vi "Configure Modules from Hardware.vi"() -> ()   [LabVIEW 2017, in "SLSC Switch Examples.lvlib"]
uses:
  SLSC Switch Examples.lvlib
  NationalInstruments.VeriStand.SystemDefinitionAPI
  SLSC Switch/Shared/Endpoint Configuration Cluster.ctl
  SLSC Switch/Shared/Endpoint Configuration Enum.ctl
  SLSC Switch/Scripting/SLSC Switch Scripting.lvlib
  SLSC Switch/Shared/SLSC Switch Shared.lvlib
panel:
  in  "SLSC Switch devices":refnum<k21>[](array[refnum])
  out "error out":errorcluster
  in  "error in (no error)":errorcluster
  in  "output system definition":path
  in  "input system definition":path
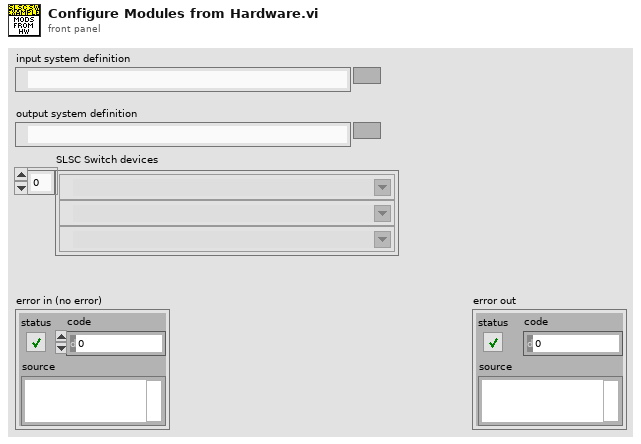
[diagram p1: front panel]
types:
  T1 = typedef "SLSC Switch Shared.lvlib/Endpoint Configuration Enum.ctl" = enum16{"Load", "Source", "Configuration"}
  T2 = typedef "SLSC Switch Shared.lvlib/Endpoint Configuration Cluster.ctl" = cluster{"Endpoint":string, "Configuration":T1}
  T3 = typedef "Custom Device API.lvlib/Custom Device Item Ref.ctl" = u64
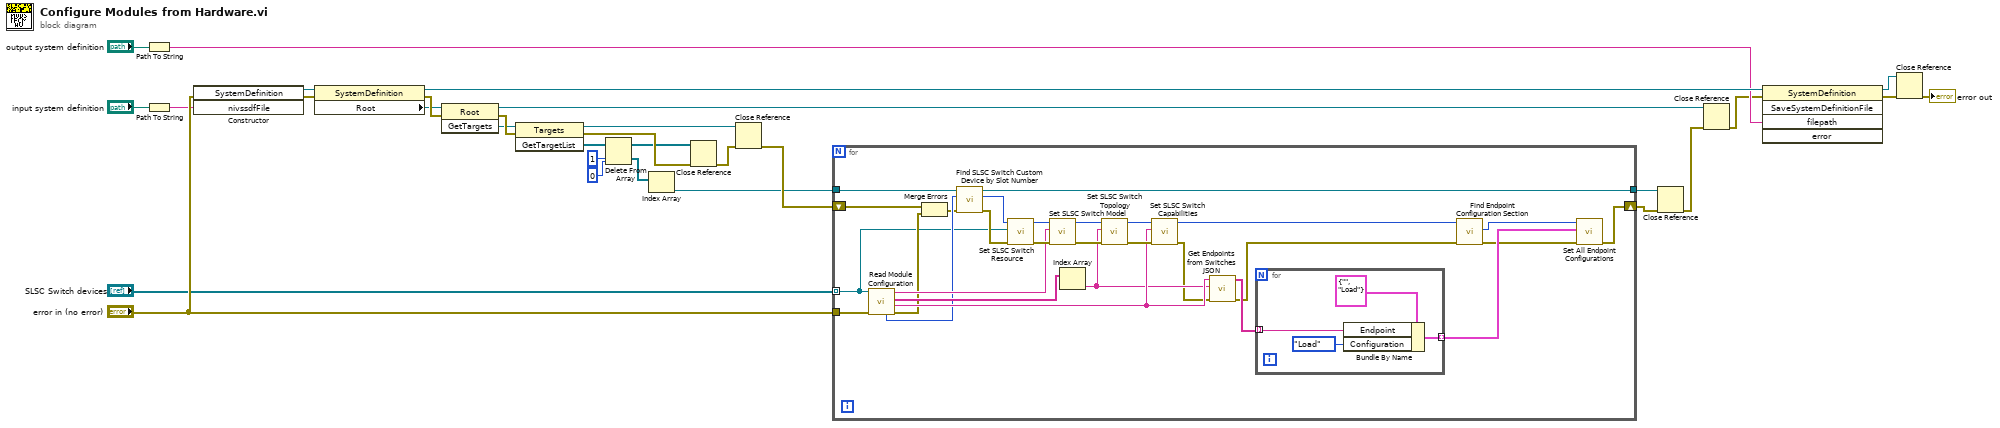
[diagram p0: block diagram]
diagram:
  n1 = Path To String(path="output system definition") -> (string=w16:string)
  n2 = Path To String(path="input system definition") -> (string=w8:string)
  n3 = constructor class="SystemDefinition"(error in="error in (no error)", "nivssdfFile"=w8) -> (reference out=w30:refnum<k24>, error out=w31:errorcluster)  [unwired: 2 in, 2 out]
  n4 = property class="SystemDefinition"(reference=w30, error in=w31) -> (reference out=w17:refnum<k24>, error out=w29:errorcluster, "Root"=w28:refnum<k24>)
  n5 = invoke class="Root" method="GetTargets"(reference=w28, error in=w29) -> (reference out=w13:refnum<k24>, error out=w27:errorcluster, "GetTargets"=w26:refnum<k24>)  [unwired: 1 in]
  n6 = invoke class="Targets" method="GetTargetList"(reference=w26, error in=w27) -> (reference out=w19:refnum<k24>, error out=w22:errorcluster, "GetTargetList"=w25:refnum<k24>[])  [unwired: 1 in]
  n7 = Delete From Array(array=w25, length=1, index=0) -> (deleted portion=w18:refnum<k24>[], array with subset deleted=w21:refnum<k24>[])
  n8 = Index Array(array=w18) -> (element=w5:refnum<k24>)  [unwired: 1 in]
  n9 = Close Reference(reference=w21, error in (no error)=w22) -> (error out=w20:errorcluster)
  n10 = Close Reference(reference=w19, error in (no error)=w20) -> (error out=w6:errorcluster)
  n11 = for {
    tunnel: "error in (no error)" -> [w46]
    tunnel: w5 -> [w44]
    tunnel: "SLSC Switch devices" -> [w34] mode=indexing
    shift-right: [w32] -> w1
    shift-left: w6 -> [w45]
    tunnel: [w33] -> w3
    n12 = call "Read Module Configuration.vi"("error in (no error)"=w46, "SLSC Device"=w34) -> ("error out"=w39:errorcluster, "switches json"=w51:string, "topologies"=w53:string[], "product name"=w57:string, "slot number"=w41:u32)  [unwired: 5 in]
    n13 = Merge Errors(w45, w39) -> (w40:errorcluster)
    n14 = call "Find SLSC Switch Custom Device by Slot Number.vi"("error in (no error)"=w40, "slot number"=w41, "Target in"=w44) -> ("error out"=w42:errorcluster, "SLSC Switch Custom Device Ref"=w43:T3, "Target out"=w33:refnum<k24>)  [unwired: 6 in]
    n15 = call "Set SLSC Switch Resource.vi"("error in (no error)"=w42, "Resource"=w34, "SLSC Switch Custom Device Ref in"=w43) -> ("error out"=w58:errorcluster, "SLSC Switch Custom Device Ref out"=w59:T3)  [unwired: 7 in]
    n16 = call "Set SLSC Switch Model.vi"("error in (no error)"=w58, "Model"=w57, "SLSC Switch Custom Device Ref in"=w59) -> ("error out"=w52:errorcluster, "SLSC Switch Custom Device Ref out"=w56:T3)  [unwired: 7 in]
    n17 = Index Array(array=w53) -> (element=w50:string)  [unwired: 1 in]
    n18 = call "Set SLSC Switch Topology.vi"("error in (no error)"=w52, "Topology"=w50, "SLSC Switch Custom Device Ref in"=w56) -> ("error out"=w54:errorcluster, "SLSC Switch Custom Device Ref out"=w55:T3)  [unwired: 7 in]
    n19 = call "Set SLSC Switch Capabilities.vi"("error in (no error)"=w54, "Capabilities"=w51, "SLSC Switch Custom Device Ref in"=w55) -> ("error out"=w49:errorcluster, "SLSC Switch Custom Device Ref out"=w37:T3)  [unwired: 7 in]
    n20 = call "Get Endpoints from Switches JSON.vi"("error in (no error)"=w49, "topology"=w50, "switches json"=w51) -> ("error out"=w38:errorcluster, "endpoints"=w48:string[])  [unwired: 7 in]
    n21 = for {
      tunnel: w48 -> [w62] mode=indexing
      tunnel: [w60] -> w47 mode=indexing
      n22 = Bundle By Name(cluster=T2 {"Endpoint"="", "Configuration"=enum."Load"} ("All Endpoint Configurations"), "Endpoint"=w62, "Configuration"=Endpoint_Configuration_Enum."Load") -> (w60:T2)
    }
    n23 = call "Find Endpoint Configuration Section.vi"("error in (no error)"=w38, "SLSC Switch Custom Device Ref in"=w37) -> ("error out"=w35:errorcluster, "Endpoint Config Section Ref"=w36:T3)  [unwired: 7 in, 1 out]
    n24 = call "Set All Endpoint Configurations.vi"("error in (no error)"=w35, "All Endpoint Configurations"=w47, "Endpoint Configuration Section Ref in"=w36) -> ("error out"=w32:errorcluster)  [unwired: 7 in, 1 out]
  }
  n25 = Close Reference(reference=w3, error in (no error)=w1) -> (error out=w2:errorcluster)
  n26 = Close Reference(reference=w13, error in (no error)=w2) -> (error out=w12:errorcluster)
  n27 = invoke class="SystemDefinition" method="SaveSystemDefinitionFile"(reference=w17, error in=w12, "filepath"=w16) -> (reference out=w14:refnum<k24>, error out=w15:errorcluster)  [unwired: 2 in, 3 out]
  n28 = Close Reference(reference=w14, error in (no error)=w15) -> (error out=→"error out":errorcluster)
